vi "Programm.vi"() -> ()   [LabVIEW 2010]
doc: "Geschwindigkeits- und Abstandsregelung \nAbschlussprojekt ELE10 Friedrich;Kauth;Schmitz\nBalthasar-Neumann-Technikum Trier"
uses:
  <vilib>/express/express arith-compare/Formula/XNode/ExpressFormulaBlockNode.xnode
  <vilib>/printing/EasyPrintingControls.llb/contents.ctl
  <vilib>/printing/EasyPrintingControls.llb/report_type.ctl
  <vilib>/printing/EasyPrinting.llb/Easy Print VI Panel or Documentation (path).vi
  <vilib>/Utility/NIReport.llb/NI_ReportGenerationCore.lvlib
panel:
  in  "Programm\nPlay/Pause":bool
  in  "Sprung \nAbstand":bool
  in  "Sprung \nGeschwin":bool
  out "Fehler (Ausgang)":errorcluster caption="Fehler"
  in  "Drucken":bool
  in  "Excel Export":bool
  out "Boolesch":bool
  in  "HILFE \nAnzeigen":bool
  out "1/x":dbl=inf caption="Tn"
  out "Tn":dbl=5.0
  in  "REG + w":bool
  in  "REG + w":bool
  in  "Ki Abstand":dbl min=0.0 step=0.1 format="%_5g"
  in  "Kp Abstand":dbl min=0.0 step=0.1 format="%_5g"
  in  "Ki Geschw.":dbl min=0.0 step=0.1 format="%_5g"
  in  "Kp Geschw.":dbl min=0.0 step=0.1 format="%_5g"
  in  "Registerkarte":T1(tab)
  out "Geschwindigkeit":dynamicdata(graph)=[{"t0"=timestamp(3419069489.296875 s since 1904-01-01), "dt"=1.0, "Y"=[0.0]}, {"t0"=timestamp(3419069489.296875 s since 1904-01-01), "dt"=1.0, "Y"=[-0.0415835524370232]}, {"t0"=timestamp(3419069489.296875 s since 1904-01-01), "dt"=1.0, "Y"=[0.0]}, {"t0"=timestamp(3419069489.296875 s since 1904-01-01), "dt"=1.0, "Y"=[0.0415835524370232]}]
  out "Abstand":dynamicdata(graph)=[{"t0"=timestamp(3419069489.296875 s since 1904-01-01), "dt"=1.0, "Y"=[0.0]}, {"t0"=timestamp(3419069489.296875 s since 1904-01-01), "dt"=1.0, "Y"=[2.3711805979498393]}, {"t0"=timestamp(3419069489.296875 s since 1904-01-01), "dt"=1.0, "Y"=[0.0]}, {"t0"=timestamp(3419069489.296875 s since 1904-01-01), "dt"=1.0, "Y"=[-2.3711805979498393]}]
  in  "w":bool=TRUE
  in  "e":bool=TRUE
  in  "y":bool=TRUE
  in  "r":bool=TRUE
  in  "w 2":bool=TRUE
  in  "r 2":bool=TRUE
  in  "e 2":bool=TRUE
  in  "y 2":bool=TRUE
  out "Geschwindigkeit \nBand in m/s":cluster{dbl, dbl}(knob)={0.0, -0.010887700107899223} scale=0.0..5.0
  out "Abstand in mm":cluster{dbl, dbl}(slide)={735.0173581435113, 901.0} scale=900.0..200.0
  out "v Auto 1":dbl(knob)=-0.010887700107899223 scale=0.0..5.0
  out "v Auto 2":dbl(knob)=-0.00855718399291744 scale=0.0..5.0
  out "OPV OUT\nGeschwindigkeit":dbl=0.3434563279828049
  out "Rückführungsgröße\nGeschwindigkeit":dbl=-0.0034129888041329708 format="%.4f"
  out "Führungsgröße\nGeschwindigkeit":dbl=1.4165304491948392 format="%.4f"
  out "Output LV\nAbstand":dbl caption="output value LV2" format="%0.2f"
  out "Output LV\nGeschwindigkeit":dbl format="%0.2f"
  out "OPV OUT\nAbstand":dbl=0.017239803538601967
  out "Rückführgröße \nAbstand":dbl=2.360986790064136
  out "Führungsgröße \nAbstand":dbl=1.403589268719555
  out "Auto 2 \nGeschwindigkeit":dbl=-0.003230257411863193
  out "Reserve AI":dbl=1.4029034874114228
  out "Numerisch":dbl
  out "Numerisch 2":dbl=-0.0415835524370232
  out "Numerisch 3":dbl
  out "Numerisch 4":dbl=0.0415835524370232
  out "Numerisch 5":dbl
  out "Numerisch 6":dbl=2.360986790064136
  out "Numerisch 7":dbl
  out "Numerisch 8":dbl=-2.360986790064136
  out "Anlage EIN":bool=TRUE
  out "OPV":bool
  out "LV":bool=TRUE
  in  "Führungsgröße \nAbstand LV":dbl min=0.0 max=10.0 step=0.1 format="%_5g"
  in  "Führungsgröße \nGeschwindigkeit LV":dbl min=0.0 max=10.0 step=0.1 format="%_5g"
  in  "Programm Stopp":bool
  # "Info USB 6008"
  # "V"
  # "V"
  # "V"
  # "V"
  # "-B3"
  # "V"
  # "-M4"
  # "-M3"
  # "-M2"
  # "V"
  # "V"
  # "V"
  # "V"
  # "M1"
  # "V"
  # "Geschwindigkeit"
  # "Abstand"
  # "V"
  # "V"
  # "V"
  # "V"
  # "V"
  # "V"
  # "V"
  # "V"
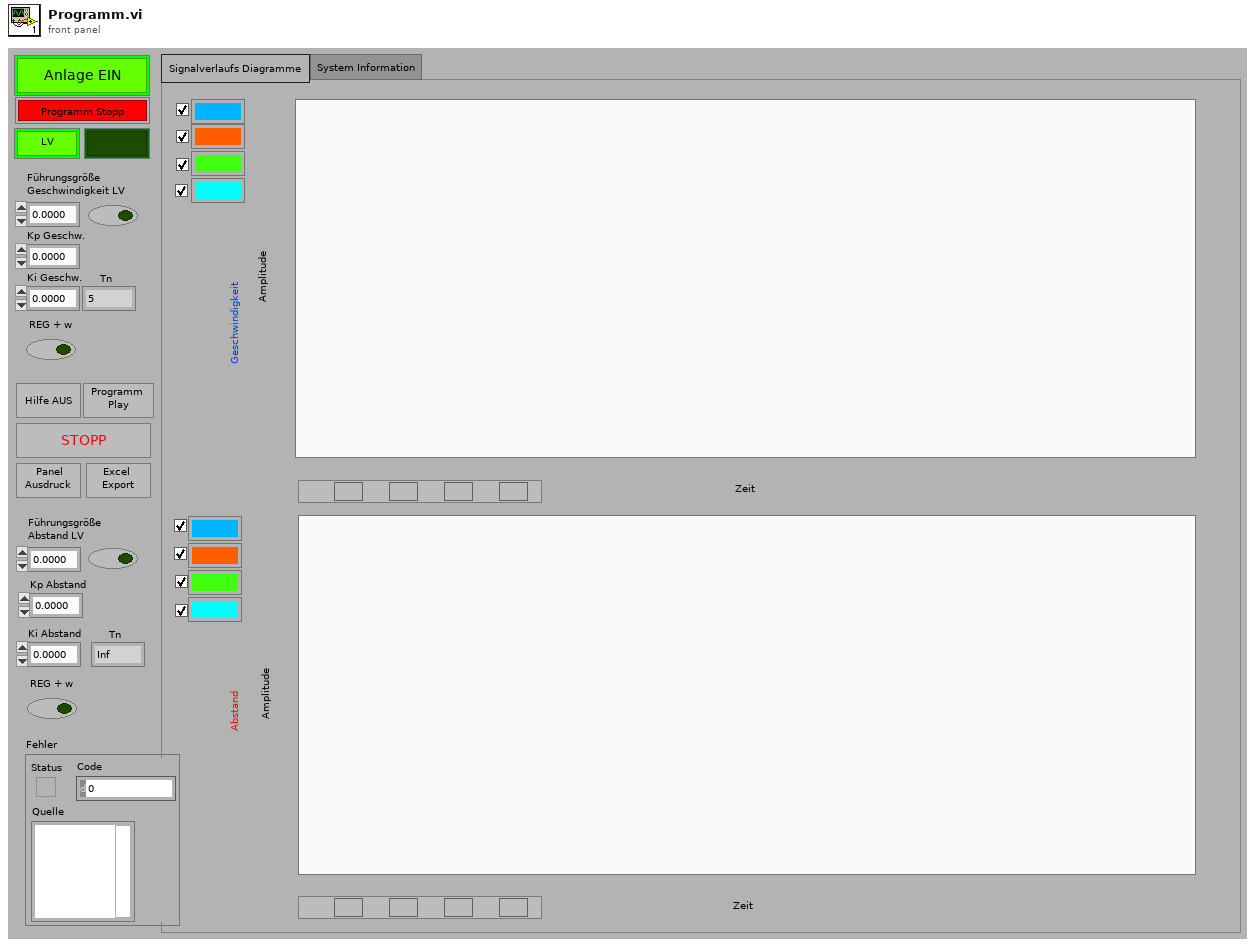
[diagram p1: front panel]
types:
  T1 = enum32{"Signalverlaufs Diagramme ", "System Information"}
  T2 = cluster{"data[0]":bool, "data[1]":bool, "data[2]":bool, "data[3]":bool, "data[4]":bool, "data[5]":bool, "data[6]":bool, "data[7]":bool, "data[8]":bool}
  T3 = enum8{"Enabled", "Disabled", "Disabled and Grayed Out"}
  T4 = typedef "NI_ReportGenerationCore.lvlib/contents.ctl" = u16
  T5 = typedef "NI_ReportGenerationCore.lvlib/report_type.ctl" = u16
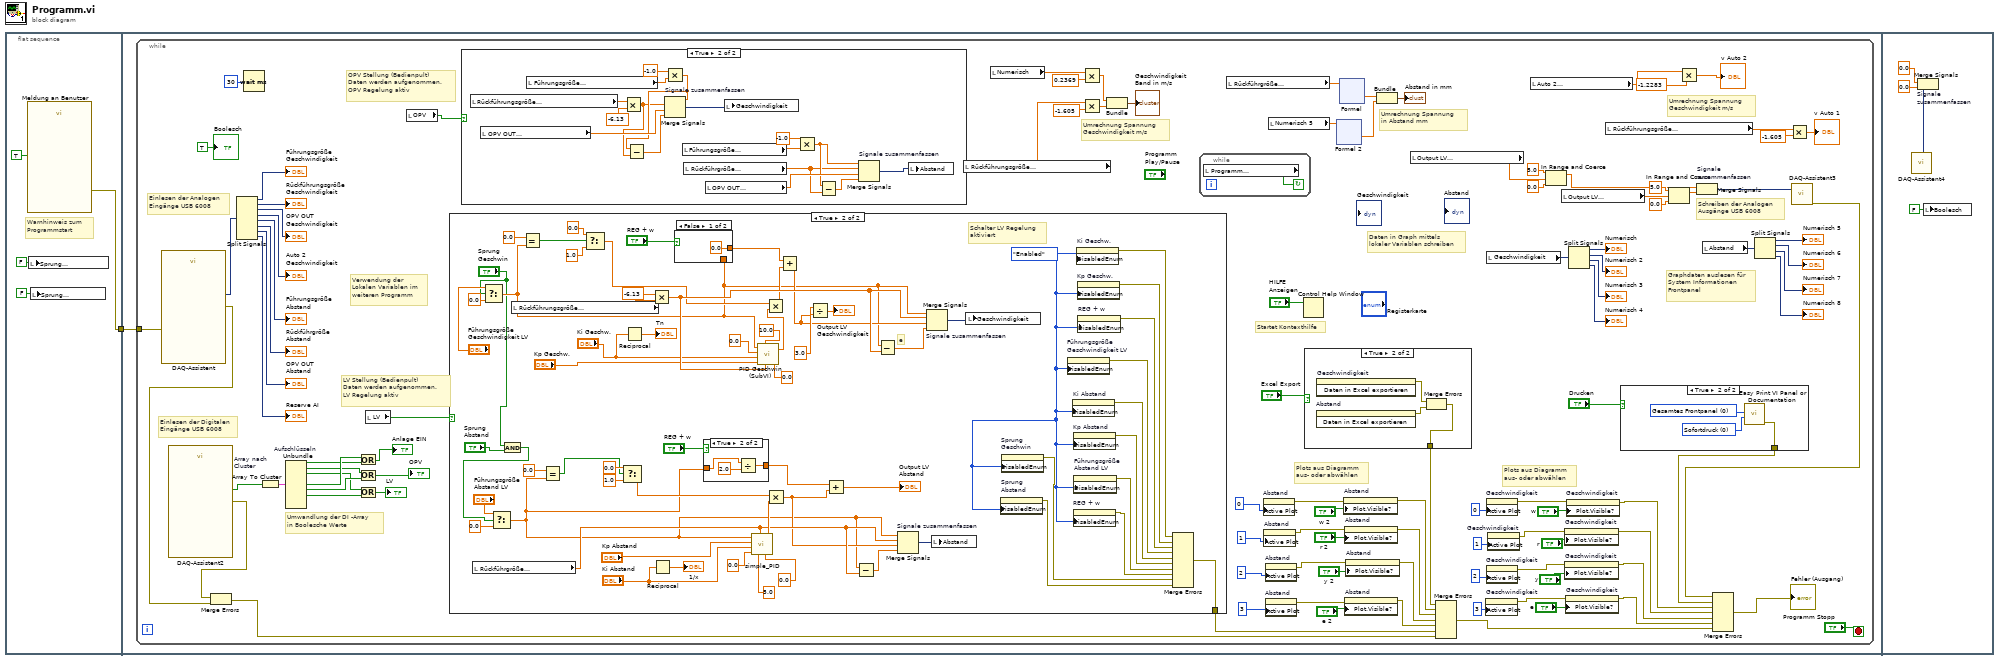
[diagram p0: block diagram]
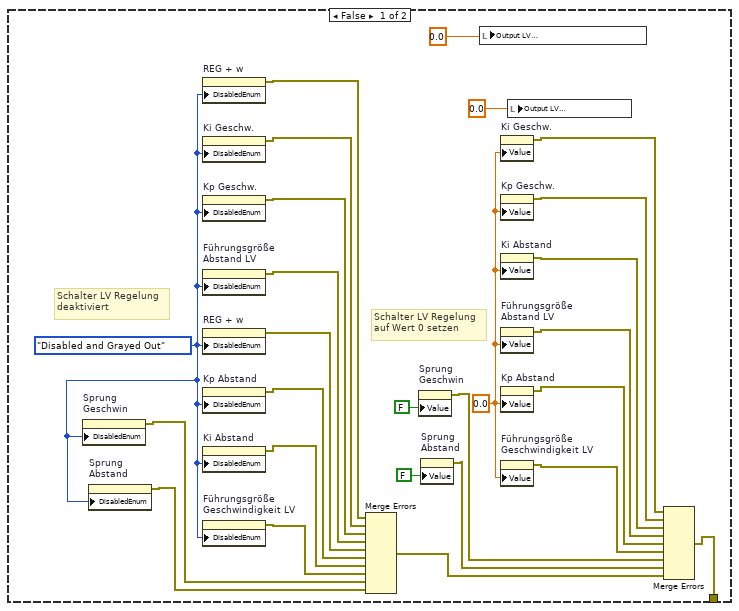
[diagram p4: hidden frame]
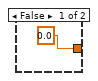
[diagram p5: hidden frame]
diagram:
  n1 = flat-sequence {
    tunnel: [w4] -> w1
    tunnel: w1 -> [w6]
    frame #0 {
      # "Warnhinweis zum \nProgrammstart"
      n2 = call "Meldung an Benutzer"("Enable"=TRUE) -> ("error out"=w4:errorcluster)  [unwired: 9 in, 1 out]
      n3 = local write "Sprung \nGeschwin"(FALSE ("Sprung \nGeschwin")) -> ()
      n4 = local write "Sprung \nAbstand"(FALSE ("Sprung \nAbstand")) -> ()
    }
    frame #1 {
      n5 = while {
        tunnel: w6 -> [w31]
        stop <- "Programm Stopp" stop-if-true
        # "Daten in Graph mittels\nlokaler Variablen schreiben"
        # "Plots aus Diagramm\naus- oder abwählen"
        # "LV Stellung (Bedienpult)\nDaten werden aufgenommen.\nLV Regelung aktiv"
        # "OPV Stellung (Bedienpult)\nDaten werden aufgenommen.\nOPV Regelung aktiv"
        # "Verwendung der \nLokalen Variablen im\nweiteren Programm"
        # "Plots aus Diagramm\naus- oder abwählen"
        # "Umrechnung Spannung\nGeschwindigkeit m/s"
        # "Umrechnung Spannung\nGeschwindigkeit m/s"
        # "Umrechnung Spannung\nin Abstand mm"
        # "Startet Kontexthilfe"
        # "Graphdaten auslesen für\nSystem Informationen \nFrontpanel"
        # "Schreiben der Analogen\nAusgänge USB 6008"
        # "Umwandlung der DI -Array\nin Boolesche Werte"
        # "Einlesen der Digitalen\nEingänge USB 6008"
        # "Einlesen der Analogen\nEingänge USB 6008"
        n6 = call "DAQ-Assistent"("error in"=w31) -> ("data"=w113:dynamicdata, "error out"=w30:errorcluster)  [unwired: 16 in, 1 out]
        n7 = call "DAQ-Assistent2"() -> ("data"=w104:bool[], "error out"=w29:errorcluster)  [unwired: 17 in, 1 out]
        n8 = Merge Errors(w29, w30) -> (w18:errorcluster)
        n9 = Split Signals(w113) -> (→"Führungsgröße\nGeschwindigkeit":dynamicdata, →"Rückführungsgröße\nGeschwindigkeit":dynamicdata, →"OPV OUT\nGeschwindigkeit":dynamicdata, →"Auto 2 \nGeschwindigkeit":dynamicdata, →"Führungsgröße \nAbstand":dynamicdata, →"Rückführgröße \nAbstand":dynamicdata, →"OPV OUT\nAbstand":dynamicdata, →"Reserve AI":dynamicdata)  [unwired: 8 in]
        n10 = Wait (ms)(milliseconds to wait=u32 30 ("Zu wartende ms")) -> ()  [unwired: 1 out]
        n11 = Array To Cluster "Array nach \nCluster"(array=w104) -> (cluster=w103:T2)
        n12 = Unbundle "Aufschlüsseln"(w103) -> ("data[0]"=w97:bool, "data[1]"=w96:bool, "data[2]"=w94:bool, "data[4]"=w98:bool, "data[5]"=w95:bool, "data[6]"=w93:bool)  [unwired: 3 out]
        n13 = Or(x=w98, y=w97) -> (x .or. y?=→"Anlage EIN":bool)
        n14 = Or(x=w96, y=w95) -> (x .or. y?=→"OPV":bool)
        n15 = Or(x=w94, y=w93) -> (x .or. y?=→"LV":bool)
        n16 = local read "LV"() -> (w83:bool)
        n17 = local read "OPV"() -> (w8:bool)
        n18 = case shown="True" w83 {
          tunnel: [w145 w177] -> w19
          frame False {
            w160 = 0.0 ("Ki Geschw.")
            w144 = T3."Disabled and Grayed Out" ("Deaktiviert")
            # "Schalter LV Regelung\nauf Wert 0 setzen"
            # "Schalter LV Regelung\ndeaktiviert"
            n19 = property on="Sprung \nGeschwin" class="Bool. (strikt)"("DisabledEnum"=w144) -> (error out=w143:errorcluster)  [unwired: 2 in, 1 out]
            n20 = property on="Sprung \nAbstand" class="Bool. (strikt)"("DisabledEnum"=w144) -> (error out=w142:errorcluster)  [unwired: 2 in, 1 out]
            n21 = property on="REG + w" class="Bool. (strikt)"("DisabledEnum"=w144) -> (error out=w153:errorcluster)  [unwired: 2 in, 1 out]
            n22 = property on="Ki Geschw." class="DigWert (strikt)"("DisabledEnum"=w144) -> (error out=w152:errorcluster)  [unwired: 2 in, 1 out]
            n23 = property on="Kp Geschw." class="DigWert (strikt)"("DisabledEnum"=w144) -> (error out=w151:errorcluster)  [unwired: 2 in, 1 out]
            n24 = property on="Führungsgröße \nAbstand LV" class="DigWert (strikt)"("DisabledEnum"=w144) -> (error out=w150:errorcluster)  [unwired: 2 in, 1 out]
            n25 = property on="REG + w" class="Bool. (strikt)"("DisabledEnum"=w144) -> (error out=w149:errorcluster)  [unwired: 2 in, 1 out]
            n26 = property on="Kp Abstand" class="DigWert (strikt)"("DisabledEnum"=w144) -> (error out=w148:errorcluster)  [unwired: 2 in, 1 out]
            n27 = property on="Ki Abstand" class="DigWert (strikt)"("DisabledEnum"=w144) -> (error out=w147:errorcluster)  [unwired: 2 in, 1 out]
            n28 = property on="Führungsgröße \nGeschwindigkeit LV" class="DigWert (strikt)"("DisabledEnum"=w144) -> (error out=w146:errorcluster)  [unwired: 2 in, 1 out]
            n29 = Merge Errors(w153, w152, w151, w150, w149, w148, w147, w146, w143, w142) -> (w137:errorcluster)
            n30 = property on="Sprung \nGeschwin" class="Bool. (strikt)"("Value"=FALSE ("Sprung \nGeschwin")) -> (error out=w139:errorcluster)  [unwired: 2 in, 1 out]
            n31 = property on="Sprung \nAbstand" class="Bool. (strikt)"("Value"=FALSE ("Sprung \nAbstand")) -> (error out=w138:errorcluster)  [unwired: 2 in, 1 out]
            n32 = local write "Output LV\nGeschwindigkeit"(0.0 ("LV OUT \nAbstand")) -> ()
            n33 = property on="Ki Geschw." class="DigWert (strikt)"("Value"=w160) -> (error out=w159:errorcluster)  [unwired: 2 in, 1 out]
            n34 = property on="Kp Geschw." class="DigWert (strikt)"("Value"=w160) -> (error out=w158:errorcluster)  [unwired: 2 in, 1 out]
            n35 = property on="Ki Abstand" class="DigWert (strikt)"("Value"=w160) -> (error out=w157:errorcluster)  [unwired: 2 in, 1 out]
            n36 = property on="Führungsgröße \nAbstand LV" class="DigWert (strikt)"("Value"=w160) -> (error out=w156:errorcluster)  [unwired: 2 in, 1 out]
            n37 = property on="Kp Abstand" class="DigWert (strikt)"("Value"=w160) -> (error out=w155:errorcluster)  [unwired: 2 in, 1 out]
            n38 = property on="Führungsgröße \nGeschwindigkeit LV" class="DigWert (strikt)"("Value"=w160) -> (error out=w154:errorcluster)  [unwired: 2 in, 1 out]
            n39 = local write "Output LV\nAbstand"(0.0 ("LV OUT\nGeschwindgkeit")) -> ()
            n40 = Merge Errors(w159, w158, w157, w156, w155, w154, w139, w138, w137) -> (w145:errorcluster)
          }
          frame True {
            w165 = T3."Enabled" ("Deaktiviert")
            # "Schalter LV Regelung\naktiviert"
            # "e"
            n41 = local read "Rückführgröße \nAbstand"() -> (w205:dbl)
            n42 = Select(t="Führungsgröße \nGeschwindigkeit LV", s="Sprung \nGeschwin", f=0.0) -> (s? t:f=w171:dbl)
            n43 = And(x="Sprung \nGeschwin", y="Sprung \nAbstand") -> (x .and. y?=w166:bool)
            n44 = Select(t="Führungsgröße \nAbstand LV", s=w166, f=0.0) -> (s? t:f=w174:dbl)
            n45 = local read "Rückführungsgröße\nGeschwindigkeit"() -> (w222:dbl)
            n46 = Equal?(x=0.0, y=w171) -> (x = y?=w176:bool)
            n47 = Equal?(x=0.0, y=w174) -> (x = y?=w175:bool)
            n48 = Select(t=0.0, s=w176, f=1.0) -> (s? t:f=w197:dbl)
            n49 = Select(t=0.0, s=w175, f=1.0) -> (s? t:f=w221:dbl)
            n50 = Reciprocal(x="Ki Geschw.") -> (1/x=→"Tn":dbl)
            n51 = Multiply(x=-6.13, y=w222) -> (x*y=w210:dbl)
            n52 = Reciprocal(x="Ki Abstand") -> (1/x=→"1/x":dbl)
            n53 = case shown="False" "REG + w" {
              tunnel: [0.0 ("Führungsgröße \nGeschwindigkeit LV") w231] -> w195
              tunnel: w171 -> [_ w231]
              frame False {
              }
              frame True {
              }
            }
            n54 = case shown="True" "REG + w" {
              tunnel: [0.0 ("Führungsgröße \nGeschwindigkeit LV") w228] -> w191
              tunnel: w174 -> [_ w227]
              frame False {
              }
              frame True {
                n55 = Divide(x=w227, y=2.0) -> (x/y=w228:dbl)
              }
            }
            n56 = call "simple_PID.vi"("lower limit"=0.0, "upper limit"=5.0, "process variable"=w205, "D"=0.0, "I"="Ki Abstand", "P"="Kp Abstand", "set point"=w174) -> ("output value"=w207:dbl)  [unwired: 4 in]
            n57 = call "PID Geschwin (SubVI).vi"("lower limit"=0.0, "Rück Geschwin"=w210, "upper limit"=10.0, "Kp Geschwin"="Kp Geschw.", "Ki Geschwin"="Ki Geschw.", "D"=0.0, "Führung Geschwin"=w171) -> ("OUT Gesch"=w206:dbl)
            n58 = Multiply(x=w197, y=w206) -> (x*y=w199:dbl)
            n59 = Multiply(x=w221, y=w207) -> (x*y=w192:dbl)
            n60 = Add(x=w195, y=w199) -> (x+y=w198:dbl)
            n61 = Divide(x=w198, y=3.0) -> (x/y=→"Output LV\nGeschwindigkeit":dbl)
            n62 = Add(x=w191, y=w192) -> (x+y=→"Output LV\nAbstand":dbl)
            n63 = Subtract(x=w174, y=w205) -> (x-y=w224:dbl)
            n64 = Subtract(x=w171, y=w210) -> (x-y=w225:dbl)
            n65 = Merge Signals "Signale zusammenfassen"(w174, w205, w192, w224) -> (w223:dynamicdata)
            n66 = Merge Signals "Signale zusammenfassen"(w171, w210, w198, w225) -> (w204:dynamicdata)
            n67 = local write "Abstand"(w223) -> ()
            n68 = local write "Geschwindigkeit"(w204) -> ()
            n69 = property on="Sprung \nAbstand" class="Bool. (strikt)"("DisabledEnum"=w165) -> (error out=w163:errorcluster)  [unwired: 2 in, 1 out]
            n70 = property on="Sprung \nGeschwin" class="Bool. (strikt)"("DisabledEnum"=w165) -> (error out=w164:errorcluster)  [unwired: 2 in, 1 out]
            n71 = property on="Führungsgröße \nGeschwindigkeit LV" class="DigWert (strikt)"("DisabledEnum"=w165) -> (error out=w182:errorcluster)  [unwired: 2 in, 1 out]
            n72 = property on="Ki Abstand" class="DigWert (strikt)"("DisabledEnum"=w165) -> (error out=w181:errorcluster)  [unwired: 2 in, 1 out]
            n73 = property on="Kp Abstand" class="DigWert (strikt)"("DisabledEnum"=w165) -> (error out=w180:errorcluster)  [unwired: 2 in, 1 out]
            n74 = property on="REG + w" class="Bool. (strikt)"("DisabledEnum"=w165) -> (error out=w178:errorcluster)  [unwired: 2 in, 1 out]
            n75 = property on="Führungsgröße \nAbstand LV" class="DigWert (strikt)"("DisabledEnum"=w165) -> (error out=w179:errorcluster)  [unwired: 2 in, 1 out]
            n76 = property on="Ki Geschw." class="DigWert (strikt)"("DisabledEnum"=w165) -> (error out=w185:errorcluster)  [unwired: 2 in, 1 out]
            n77 = property on="Kp Geschw." class="DigWert (strikt)"("DisabledEnum"=w165) -> (error out=w184:errorcluster)  [unwired: 2 in, 1 out]
            n78 = property on="REG + w" class="Bool. (strikt)"("DisabledEnum"=w165) -> (error out=w183:errorcluster)  [unwired: 2 in, 1 out]
            n79 = Merge Errors(w185, w184, w183, w182, w181, w180, w179, w178, w164, w163) -> (w177:errorcluster)
          }
        }
        n80 = case shown="True" w8 {
          frame False {
          }
          frame True {
            n81 = local read "Rückführungsgröße\nGeschwindigkeit"() -> (w244:dbl)
            n82 = local read "OPV OUT\nGeschwindigkeit"() -> (w247:dbl)
            n83 = local read "Führungsgröße\nGeschwindigkeit"() -> (w242:dbl)
            n84 = Multiply(x=w244, y=-6.13) -> (x*y=w236:dbl)
            n85 = Multiply(x=-1.0, y=w242) -> (x*y=w237:dbl)
            n86 = Subtract(x=w237, y=w236) -> (x-y=w235:dbl)
            n87 = Merge Signals "Signale zusammenfassen"(w237, w236, w247, w235) -> (w238:dynamicdata)
            n88 = local read "Führungsgröße \nAbstand"() -> (w240:dbl)
            n89 = local read "Rückführgröße \nAbstand"() -> (w232:dbl)
            n90 = local read "OPV OUT\nAbstand"() -> (w246:dbl)
            n91 = local write "Geschwindigkeit"(w238) -> ()
            n92 = Multiply(x=-1.0, y=w240) -> (x*y=w233:dbl)
            n93 = Subtract(x=w233, y=w232) -> (x-y=w234:dbl)
            n94 = Merge Signals "Signale zusammenfassen"(w233, w232, w246, w234) -> (w245:dynamicdata)
            n95 = local write "Abstand"(w245) -> ()
          }
        }
        n96 = local read "Rückführungsgröße\nGeschwindigkeit"() -> (w7:dbl)
        n97 = local read "Numerisch"() -> (w40:dbl)
        n98 = Multiply(x=w40, y=0.2369) -> (x*y=w38:dbl)
        n99 = Multiply(x=w7, y=-1.605) -> (x*y=w36:dbl)
        n100 = Bundle(w38, w36) -> (→"Geschwindigkeit \nBand in m/s":cluster{dbl, dbl})  [unwired: 1 in]
        n101 = while {
          stop <- w114 continue-if-true
          n102 = local read "Programm\nPlay/Pause"() -> (w114:bool)
        }
        n103 = local read "Rückführgröße \nAbstand"() -> (w48:dbl)
        n104 = property on="Abstand" class="SVDiagr (strikt)"("Active Plot"=u32 0 ("Aktiver Plot")) -> (error out=w70:errorcluster)  [unwired: 2 in, 1 out]
        n105 = property on="Abstand" class="SVDiagr (strikt)"("Active Plot"=u32 1 ("Aktiver Plot")) -> (error out=w69:errorcluster)  [unwired: 2 in, 1 out]
        n106 = property on="Abstand" class="SVDiagr (strikt)"("Active Plot"=u32 2 ("Aktiver Plot")) -> (error out=w68:errorcluster)  [unwired: 2 in, 1 out]
        n107 = property on="Abstand" class="SVDiagr (strikt)"("Active Plot"=u32 3 ("Aktiver Plot")) -> (error out=w67:errorcluster)  [unwired: 2 in, 1 out]
        n108 = local read "Numerisch 5"() -> (w41:dbl)
        n109 = Control Help Window(1:"HILFE \nAnzeigen") -> ()  [unwired: 1 in]
        n110 = case shown="True" "Excel Export" {
          tunnel: [_ w118] -> w15
          frame False {
          }
          frame True {
            n111 = invoke on="Abstand" class="SVDiagr (strikt)" method="Daten in Excel exportieren"() -> (error out=w119:errorcluster)  [unwired: 3 in, 2 out]
            n112 = invoke on="Geschwindigkeit" class="SVDiagr (strikt)" method="Daten in Excel exportieren"() -> (error out=w120:errorcluster)  [unwired: 3 in, 2 out]
            n113 = Merge Errors(w120, w119) -> (w118:errorcluster)
          }
        }
        n114 = xnode "Formel 2"("X1"=w41) -> ("Ergebnis"=w43:dbl)  [unwired: 1 in, 1 out]
        n115 = xnode "Formel"("X1"=w48) -> ("Ergebnis"=w44:dbl)  [unwired: 1 in, 1 out]
        n116 = property on="Abstand" class="SVDiagr (strikt)"(error in=w70, "Plot.Visible?"="w 2") -> (error out=w28:errorcluster)  [unwired: 1 in, 1 out]
        n117 = property on="Abstand" class="SVDiagr (strikt)"(error in=w69, "Plot.Visible?"="r 2") -> (error out=w27:errorcluster)  [unwired: 1 in, 1 out]
        n118 = property on="Abstand" class="SVDiagr (strikt)"(error in=w67, "Plot.Visible?"="e 2") -> (error out=w25:errorcluster)  [unwired: 1 in, 1 out]
        n119 = property on="Abstand" class="SVDiagr (strikt)"(error in=w68, "Plot.Visible?"="y 2") -> (error out=w26:errorcluster)  [unwired: 1 in, 1 out]
        n120 = Bundle("Ergebnis"=w44, "Ergebnis"=w43) -> (→"Abstand in mm":cluster{"Ergebnis":dbl, "Ergebnis":dbl})  [unwired: 1 in]
        n121 = local read "Output LV\nGeschwindigkeit"() -> (w90:dbl)
        n122 = Merge Errors(w15, w28, w27, w26, w25, w19, w18) -> (w20:errorcluster)
        n123 = property on="Geschwindigkeit" class="SVDiagr (strikt)"("Active Plot"=u32 3 ("Aktiver Plot")) -> (error out=w71:errorcluster)  [unwired: 2 in, 1 out]
        n124 = property on="Geschwindigkeit" class="SVDiagr (strikt)"("Active Plot"=u32 0 ("Aktiver Plot")) -> (error out=w82:errorcluster)  [unwired: 2 in, 1 out]
        n125 = property on="Geschwindigkeit" class="SVDiagr (strikt)"("Active Plot"=u32 2 ("Aktiver Plot")) -> (error out=w74:errorcluster)  [unwired: 2 in, 1 out]
        n126 = local read "Geschwindigkeit"() -> (w58:dynamicdata)
        n127 = property on="Geschwindigkeit" class="SVDiagr (strikt)"("Active Plot"=u32 1 ("Aktiver Plot")) -> (error out=w76:errorcluster)  [unwired: 2 in, 1 out]
        n128 = local read "Auto 2 \nGeschwindigkeit"() -> (w9:dbl)
        n129 = In Range and Coerce(upper limit=5.0 ("Obergrenze"), x=w90, lower limit=0.0 ("Untergrenze")) -> (coerced(x)=w85:dbl)  [unwired: 1 out]
        n130 = local read "Output LV\nAbstand"() -> (w89:dbl)
        n131 = property on="Geschwindigkeit" class="SVDiagr (strikt)"(error in=w76, "Plot.Visible?"="r") -> (error out=w23:errorcluster)  [unwired: 1 in, 1 out]
        n132 = property on="Geschwindigkeit" class="SVDiagr (strikt)"(error in=w74, "Plot.Visible?"="y") -> (error out=w22:errorcluster)  [unwired: 1 in, 1 out]
        n133 = property on="Geschwindigkeit" class="SVDiagr (strikt)"(error in=w71, "Plot.Visible?"="e") -> (error out=w21:errorcluster)  [unwired: 1 in, 1 out]
        n134 = property on="Geschwindigkeit" class="SVDiagr (strikt)"(error in=w82, "Plot.Visible?"="w") -> (error out=w24:errorcluster)  [unwired: 1 in, 1 out]
        n135 = Split Signals(w58) -> (→"Numerisch":dynamicdata, →"Numerisch 2":dynamicdata, →"Numerisch 3":dynamicdata, →"Numerisch 4":dynamicdata)  [unwired: 4 in]
        n136 = local read "Rückführungsgröße\nGeschwindigkeit"() -> (w46:dbl)
        n137 = case shown="True" "Drucken" {
          tunnel: [_ w115] -> w17
          frame False {
          }
          frame True {
            w116 = T4 0 items=["Gesamtes Frontpanel", "Sichtbarer Bereich des Frontpanels", "Symbol, Beschreibung, Panel und Diagramm", "Dokumentation: Panel verwenden", "Dokumentation: Als SubVI verwenden", "Dokumentation: Vollständig", "Dokumentation: Benutzerdefiniert"] ("contents (complete front panel)")
            w117 = T5 0 items=["Sofortdruck", "Standardprotokoll", "HTML", "Word", "Excel"] ("report type (Quick Print)")
            n138 = call-poly <vilib>:"Easy Print VI Panel or Documentation.vi"("report type (Quick Print)"=w117, "contents (complete front panel)"=w116) -> ("error out"=w115:errorcluster)  [unwired: 8 in, 1 out]
          }
        }
        n139 = In Range and Coerce(upper limit=5.0 ("Obergrenze"), x=w89, lower limit=0.0 ("Untergrenze")) -> (coerced(x)=w86:dbl)  [unwired: 1 out]
        n140 = Multiply(x=w9, y=-1.2283) -> (x*y=→"v Auto 2":dbl)
        n141 = Merge Signals "Signale \nzusammenfassen"(w85, w86) -> (w102:dynamicdata)
        n142 = local read "Abstand"() -> (w53:dynamicdata)
        n143 = Split Signals(w53) -> (→"Numerisch 5":dynamicdata, →"Numerisch 6":dynamicdata, →"Numerisch 7":dynamicdata, →"Numerisch 8":dynamicdata)  [unwired: 4 in]
        n144 = Multiply(x=w46, y=-1.605) -> (x*y=→"v Auto 1":dbl)
        n145 = call "DAQ-Assistent3"("data"=w102) -> ("error out"=w16:errorcluster)  [unwired: 17 in, 1 out]
        n146 = Merge Errors(w16, w17, w24, w23, w22, w21, w20) -> (→"Fehler (Ausgang)":errorcluster)
        "Boolesch" <- TRUE ("Boolesch")
      }
    }
    frame #2 {
      n147 = Merge Signals "Signale \nzusammenfassen"(0.0, 0.0) -> (w249:dynamicdata)
      n148 = call "DAQ-Assistent4"("data"=w249) -> ()  [unwired: 17 in, 2 out]
      n149 = local write "Boolesch"(FALSE ("Boolesch")) -> ()
    }
  }
